vi "Example Loopback - ReadCallback Callback.vi"(4 "ReadCallback":refnum<user-event>, 5 "Event Data":T1, 6 "Control Ref":refnum<k24>, 7 "Event Common Data":T2) -> ()   [LabVIEW 2013]
uses:
  C:/tf/play/labview/Tinkerforge.dll
  Tinkerforge.dll
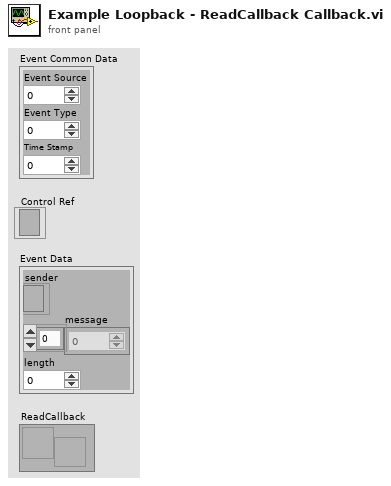
[diagram p1: front panel]
types:
  T1 = cluster{"sender":refnum<k24>, "message":u16[], "length":u8}
  T2 = cluster{"Event Source":i32, "Event Type":u32, "Time Stamp":u32}
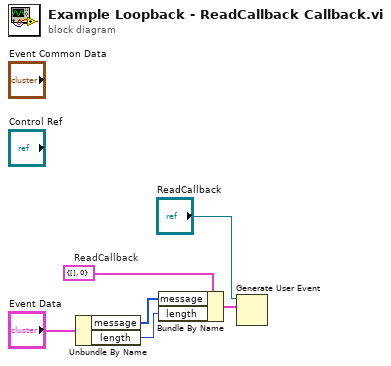
[diagram p0: block diagram]
diagram:
  w5 = cluster{"message":u16[], "length":u8} {"message"=[], "length"=0}  # ReadCallback
  n1 = Unbundle By Name("Event Data") -> ("message"=w4:u16[], "length"=w3:u8)
  n2 = Bundle By Name(cluster=w5, "message"=w4, "length"=w3) -> (w2:cluster{"message":u16[], "length":u8})
  n3 = Generate User Event(user event="ReadCallback", event data cluster=w2) -> ()  [unwired: 2 in, 2 out]
